vi "Periodic Tasks.vi"(8 "error in":errorcluster) -> ()   [LabVIEW 2012]
doc: "This VI runs in parallel to other tasks. It can contain as many user-defined periodic loops as you need. These can carry out PID or other sorts of timed response."
uses:
  <vilib>/Rock Robotics/SystemInterfaces/Utilities/FPGA_UtilitiesLED Source.ctl
  <vilib>/Rock Robotics/SystemInterfaces/Utilities/FPGA_UtilitiesLED State.ctl
  <vilib>/Rock Robotics/WPI/Solenoid/WPI_SolenoidValue.ctl
  <vilib>/Rock Robotics/WPI/RobotDrive/WPI_RobotDriveGetSetRefNum.vi
  <vilib>/Rock Robotics/WPI/Compressor/WPI_CompressorGetSetRefNum.vi
  Robot Global Data.vi
  <vilib>/Rock Robotics/WPI/Joystick/WPI_JoystickGetSetRefNum.vi
  <vilib>/Rock Robotics/WPI/Solenoid/WPI_SolenoidSetEnum.vi
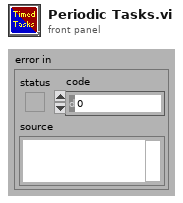
[diagram p1: front panel]
types:
  T1 = typedef "WPI_MotorControlDeviceRef.ctl" = cluster{"DeviceStatus":errorcluster, "Type":enum16{"PWM", "CAN"}, "PWM":cluster{"Digital Module":T2, "PWM Channel":T3, "DeadBand":T4}, "CAN":cluster{"Device Number":u8, "Control Mode":T5, "Semaphore":T6, "Max Vout":dbl}, "Invert":bool, "TransformRef":T7, "InvTransformRef":T7}
  T2 = typedef "FPGA_TypedefDigitalModule.ctl" = enum16{"Digital Module 1", "Digital Module 2"}
  T3 = typedef "FPGA_DIOPWMChannel.ctl" = enum8{"PWM 1", "PWM 2", "PWM 3", "PWM 4", "PWM 5", "PWM 6", "PWM 7", "PWM 8", "PWM 9", "PWM 10", "Invalid"}
  T4 = typedef "WPI_PWMDeadband.ctl" = cluster{"Name":string, "maxPositivePwm":i32, "minPositivePwm":i32, "centerPwm":i32, "maxNegativePwm":i32, "minNegativePwm":i32, "angularRange":u16}
  T5 = typedef "WPI_CANJaguar_ControlMode.ctl" = enum8{"Percent VBus", "Current", "Speed", "Position", "Voltage"}
  T6 = typedef "Semaphore RefNum" = refnum<k1>
  T7 = typedef "WPI_PWMTransform_ConPane.ctl" = refnum<vi>
  T8 = typedef "WPI_JoystickDevRef.ctl" = cluster{"Device":T9}
  T9 = typedef "WPI_JoystickDeviceEnum.ctl" = enum16{"USB 1", "USB 2", "USB 3", "USB 4", "Kinect 1", "Kinect 2"}
  T10 = typedef "WPI_JoystickButtonState.ctl" = cluster{"Button 1":bool, "Button 2":bool, "Button 3":bool, "Button 4":bool, "Button 5":bool, "Button 6":bool, "Button 7":bool, "Button 8":bool, "Button 9":bool, "Button 10":bool, "Button 11":bool, "Button 12":bool}
  T11 = cluster{"axis 1 (x)":dbl, "axis 2 (y)":dbl, "axis 3 (throttle)":dbl, "axis 4":dbl, "axis 5":dbl, "axis 6":dbl}
  T12 = typedef "WPI_SolenoidValue.ctl" = enum16{"Off", "On", "Forward", "Reverse"}
  T13 = typedef "WPI_SolenoidDevRef.ctl" = cluster{"DevStatus":errorcluster, "Solenoid Module":T14, "Forward Solenoid Channel":T15, "Reverse Solenoid Channel":T15}
  T14 = typedef "FPGA_TypedefSolenoidModule.ctl" = enum16{"Solenoid Module 1", "Solenoid Module 2"}
  T15 = typedef "WPI_SolenoidChannel.ctl" = enum8{"Solenoid 1", "Solenoid 2", "Solenoid 3", "Solenoid 4", "Solenoid 5", "Solenoid 6", "Solenoid 7", "Solenoid 8", "Invalid"}
  T16 = typedef "WPI_RobotDriveDevRef.ctl" = cluster{"DevStatus":errorcluster, "Motors[]":T1[], "Square Inputs":bool, "Max Output":dbl, "Isochronous":bool}
  T17 = typedef "WPI_CompressorDevRef.ctl" = cluster{"DevStatus":errorcluster, "DigitalInputDevRef":T18, "RelayDevRef":T20}
  T18 = typedef "WPI_DigitalInputDevRef.ctl" = cluster{"DevStatus":errorcluster, "DIO Channel":T19, "Digital Module":T2}
  T19 = typedef "FPGA_DIOChannel.ctl" = enum8{"DIO 1", "DIO 2", "DIO 3", "DIO 4", "DIO 5", "DIO 6", "DIO 7", "DIO 8", "DIO 9", "DIO 10", "DIO 11", "DIO 12", "DIO 13", "DIO 14", "Invalid"}
  T20 = typedef "WPI_RelayDevRef.ctl" = cluster{"DevStatus":errorcluster, "Relay Channel":T21, "Digital Module":T2, "Relay Direction":T22}
  T21 = typedef "FPGA_DIORelayChannel.ctl" = enum8{"Relay 1", "Relay 2", "Relay 3", "Relay 4", "Relay 5", "Relay 6", "Relay 7", "Relay 8", "Invalid"}
  T22 = typedef "WPI_RelayDirection.ctl" = enum16{"Both directions", "Forward only", "Reverse only"}
  T23 = typedef "WPI_DigitalOutputDevRef.ctl" = cluster{"Digital Module":T2, "DIO Channel":T19, "DevStatus":errorcluster}
  T24 = cluster{"JoystickDevRef":T8, "RobotDriveDevRef":T16}
  T25 = typedef "FPGA_UtilitiesLED State.ctl" = enum16{"Off", "On", "Toggle"}
  T26 = typedef "FPGA_UtilitiesLED Source.ctl" = enum16{"User LED", "FPGA LED"}
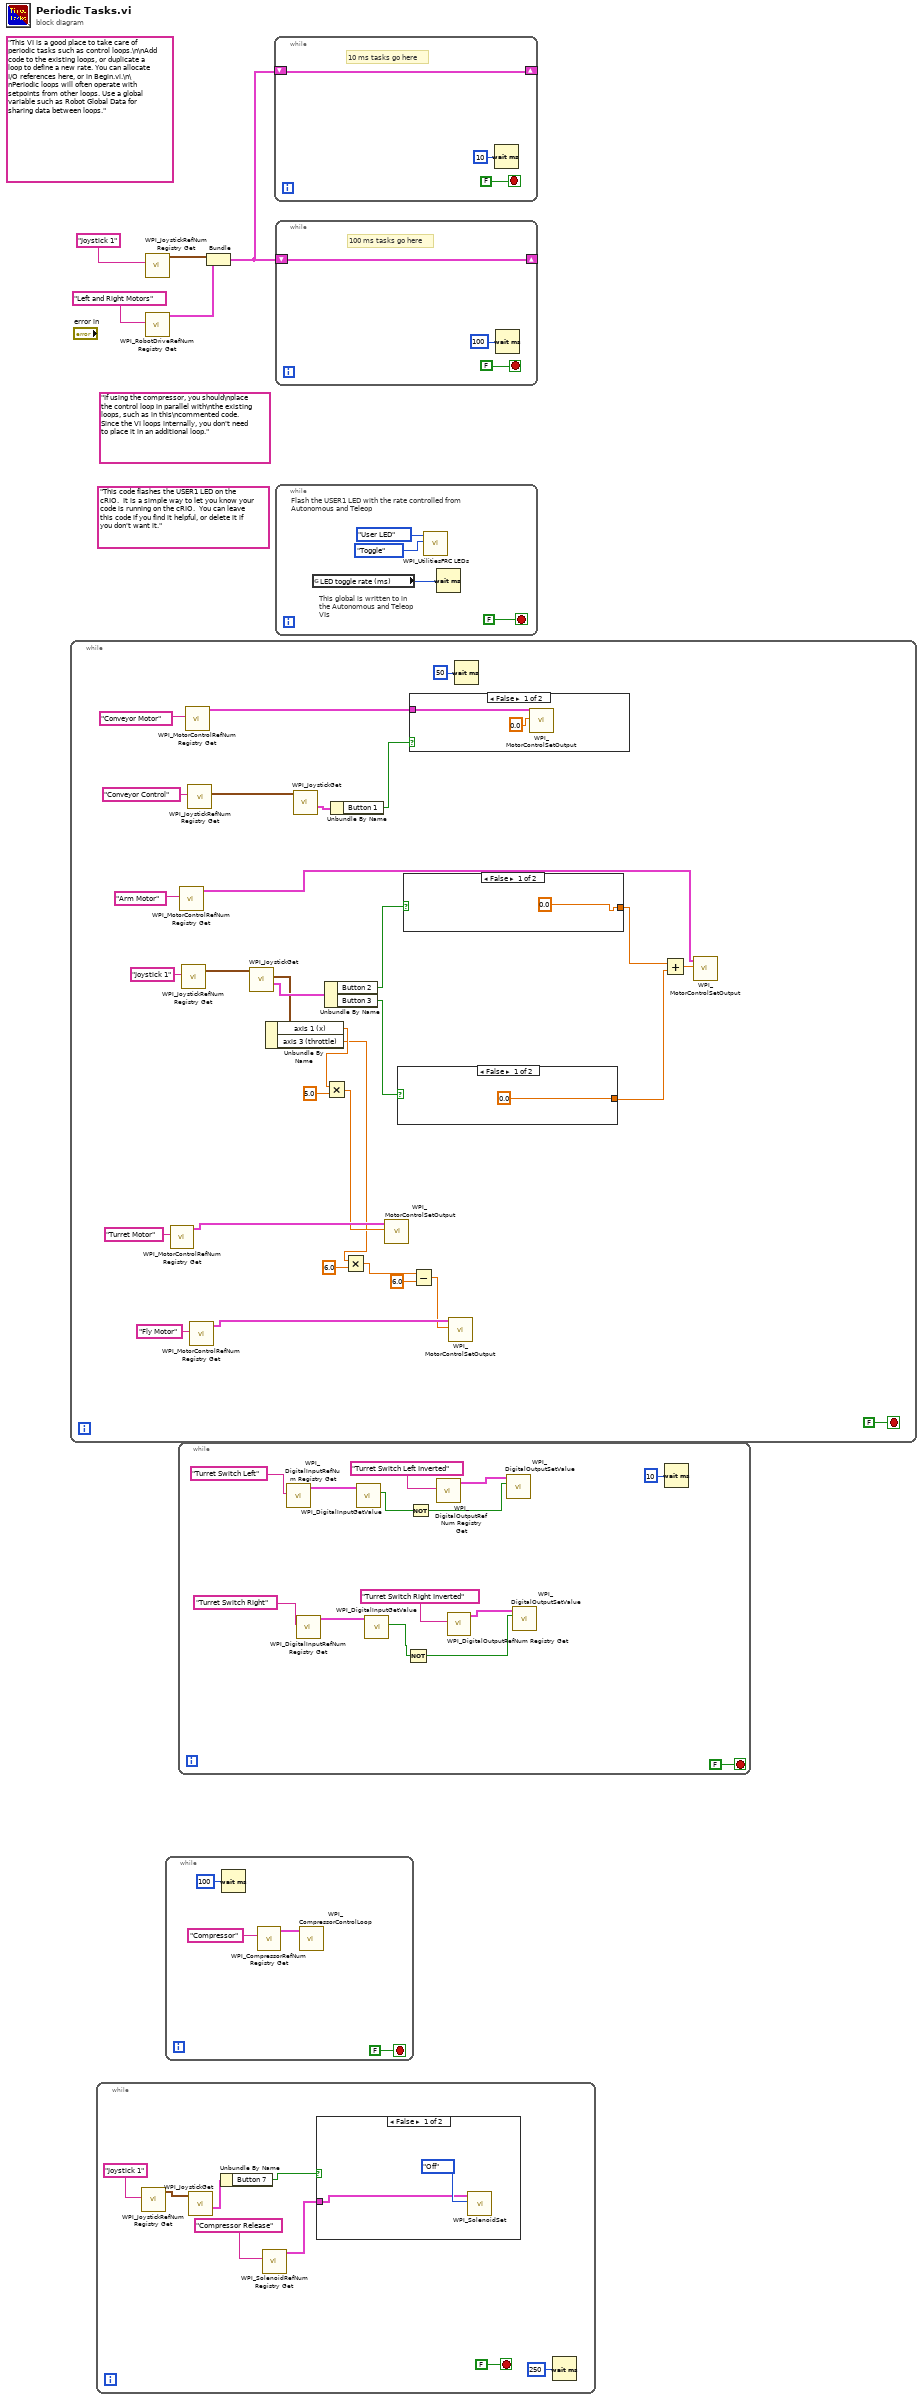
[diagram p0: block diagram]
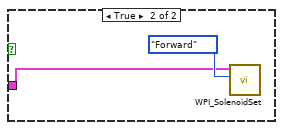
[diagram p2: hidden frame]
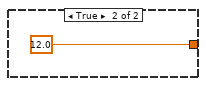
[diagram p3: hidden frame]
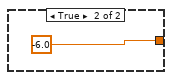
[diagram p4: hidden frame]
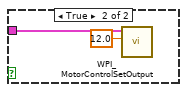
[diagram p5: hidden frame]
diagram:
  (unwired) "If using the compressor, you should\nplace the control loop in parallel with\nthe existing loops, such as in this\ncommented code. Since the VI loops internally, you don't need to place it in an additional loop."
  (unwired) "This code flashes the USER1 LED on the cRIO.  It is a simple way to let you know your code is running on the cRIO.  You can leave this code if you find it helpful, or delete it if you don't want it."
  (unwired) "This VI is a good place to take care of periodic tasks such as control loops.\n\nAdd code to the existing loops, or duplicate a loop to define a new rate. You can allocate I/O references here, or in Begin.vi.\n\nPeriodic loops will often operate with setpoints from other loops. Use a global variable such as Robot Global Data for sharing data between loops."
  n1 = while {
    stop <- FALSE stop-if-true
    n2 = call <vilib>:"WPI_MotorControlRefNum Registry Get.vi"("refnum name"="Turret Motor") -> ("MotorControlDevRef"=w20:T1)  [unwired: 9 in, 1 out]
    n3 = call <vilib>:"WPI_MotorControlRefNum Registry Get.vi"("refnum name"="Arm Motor") -> ("MotorControlDevRef"=w9:T1)  [unwired: 9 in, 1 out]
    n4 = call <vilib>:"WPI_JoystickRefNum Registry Get.vi"("refnum name"="Joystick 1") -> ("JoystickDevRef"=w26:T8)  [unwired: 9 in, 1 out]
    n5 = call <vilib>:"WPI_MotorControlRefNum Registry Get.vi"("refnum name"="Conveyor Motor") -> ("MotorControlDevRef"=w35:T1)  [unwired: 9 in, 1 out]
    n6 = call <vilib>:"WPI_JoystickRefNum Registry Get.vi"("refnum name"="Conveyor Control") -> ("JoystickDevRef"=w31:T8)  [unwired: 9 in, 1 out]
    n7 = call <vilib>:"WPI_MotorControlRefNum Registry Get.vi"("refnum name"="Fly Motor") -> ("MotorControlDevRef"=w15:T1)  [unwired: 9 in, 1 out]
    n8 = call <vilib>:"WPI_JoystickGet.vi"("JoystickDevRef"=w26) -> ("Buttons"=w25:T10, "Axes"=w21:T11)  [unwired: 4 in, 1 out]
    n9 = Unbundle By Name(w21) -> ("axis 1 (x)"=w18:dbl, "axis 3 (throttle)"=w13:dbl)
    n10 = call <vilib>:"WPI_JoystickGet.vi"("JoystickDevRef"=w31) -> ("Buttons"=w30:T10)  [unwired: 4 in, 2 out]
    n11 = Unbundle By Name(w25) -> ("Button 2"=w24:bool, "Button 3"=w23:bool)
    n12 = Multiply(x=w18, y=5.0) -> (x*y=w17:dbl)
    n13 = Unbundle By Name(w30) -> ("Button 1"=w29:bool)
    n14 = Multiply(x=w13, y=6.0) -> (x*y=w12:dbl)
    n15 = call <vilib>:"WPI_MotorControlSetOutput.vi"("Output"=w17, "MotorControlDevRef"=w20) -> ()  [unwired: 7 in, 3 out]
    n16 = case shown="False" w23 {
      tunnel: [0.0 ("Output") 12.0 ("x")] -> w6
      frame False {
      }
      frame True {
      }
    }
    n17 = case shown="False" w24 {
      tunnel: [0.0 ("x") -6.0 ("x")] -> w7
      frame False {
      }
      frame True {
      }
    }
    n18 = case shown="False" w29 {
      tunnel: w35 -> [w41 w44]
      frame False {
        n19 = call <vilib>:"WPI_MotorControlSetOutput.vi"("Output"=0.0, "MotorControlDevRef"=w41) -> ()  [unwired: 7 in, 3 out]
      }
      frame True {
        n20 = call <vilib>:"WPI_MotorControlSetOutput.vi"("Output"=12.0, "MotorControlDevRef"=w44) -> ()  [unwired: 7 in, 3 out]
      }
    }
    n21 = Subtract(x=w12, y=6.0) -> (x-y=w10:dbl)
    n22 = call <vilib>:"WPI_MotorControlSetOutput.vi"("Output"=w10, "MotorControlDevRef"=w15) -> ()  [unwired: 7 in, 3 out]
    n23 = Wait (ms)(milliseconds to wait=u32 50) -> ()  [unwired: 1 out]
    n24 = Add(x=w7, y=w6) -> (x+y=w8:dbl)
    n25 = call <vilib>:"WPI_MotorControlSetOutput.vi"("Output"=w8, "MotorControlDevRef"=w9) -> ()  [unwired: 7 in, 3 out]
  }
  n26 = while {
    stop <- FALSE stop-if-true
    n27 = call <vilib>:"WPI_JoystickRefNum Registry Get.vi"("refnum name"="Joystick 1") -> ("JoystickDevRef"=w47:T8)  [unwired: 9 in, 1 out]
    n28 = call <vilib>:"WPI_JoystickGet.vi"("JoystickDevRef"=w47) -> ("Buttons"=w46:T10)  [unwired: 4 in, 2 out]
    n29 = Unbundle By Name(w46) -> ("Button 7"=w45:bool)
    n30 = call <vilib>:"WPI_SolenoidRefNum Registry Get.vi"("refnum name"="Compressor Release") -> ("SolenoidDevRef"=w48:T13)  [unwired: 9 in, 1 out]
    n31 = case shown="False" w45 {
      tunnel: w48 -> [w53 w55]
      frame False {
        n32 = call-poly <vilib>:"WPI_SolenoidSet.vi"("Value"=WPI_SolenoidValue."Off", "SolenoidDevRef"=w53) -> ()  [unwired: 8 in, 2 out]
      }
      frame True {
        n33 = call-poly <vilib>:"WPI_SolenoidSet.vi"("Value"=WPI_SolenoidValue."Forward", "SolenoidDevRef"=w55) -> ()  [unwired: 8 in, 2 out]
      }
    }
    n34 = Wait (ms)(milliseconds to wait=u32 250) -> ()  [unwired: 1 out]
  }
  n35 = call <vilib>:"WPI_JoystickRefNum Registry Get.vi"("refnum name"="Joystick 1") -> ("JoystickDevRef"=w3:T8)  [unwired: 1 in, 9 out]
  n36 = call <vilib>:"WPI_RobotDriveRefNum Registry Get.vi"("refnum name"="Left and Right Motors") -> ("RobotDriveDevRef"=w2:T16)  [unwired: 1 in, 9 out]
  n37 = while {
    stop <- FALSE stop-if-true
    n38 = Wait (ms)(milliseconds to wait=u32 100) -> ()  [unwired: 1 out]
    n39 = call <vilib>:"WPI_CompressorRefNum Registry Get.vi"("refnum name"="Compressor") -> ("CompressorDevRef"=w60:T17)  [unwired: 9 in, 1 out]
    n40 = call <vilib>:"WPI_CompressorControlLoop.vi"("CompressorDevRef"=w60) -> ()  [unwired: 11 in]
  }
  n41 = while {
    stop <- FALSE stop-if-true
    n42 = call <vilib>:"WPI_DigitalInputRefNum Registry Get.vi"("refnum name"="Turret Switch Left") -> ("DigitalInputDevRef"=w69:T18)  [unwired: 9 in, 1 out]
    n43 = call <vilib>:"WPI_DigitalInputRefNum Registry Get.vi"("refnum name"="Turret Switch Right") -> ("DigitalInputDevRef"=w70:T18)  [unwired: 9 in, 1 out]
    n44 = call <vilib>:"WPI_DigitalInputGetValue.vi"("DigitalInputDevRef"=w69) -> ("Value"=w62:bool)  [unwired: 8 in, 2 out]
    n45 = call <vilib>:"WPI_DigitalInputGetValue.vi"("DigitalInputDevRef"=w70) -> ("Value"=w64:bool)  [unwired: 8 in, 2 out]
    n46 = Not(x=w64) -> (.not. x?=w63:bool)
    n47 = Not(x=w62) -> (.not. x?=w61:bool)
    n48 = call <vilib>:"WPI_DigitalOutputRefNum Registry Get.vi"("refnum name"="Turret Switch Left Inverted") -> ("DigitalOutputDevRef"=w65:T23)  [unwired: 9 in, 1 out]
    n49 = call <vilib>:"WPI_DigitalOutputRefNum Registry Get.vi"("refnum name"="Turret Switch Right Inverted") -> ("DigitalOutputDevRef"=w66:T23)  [unwired: 9 in, 1 out]
    n50 = call <vilib>:"WPI_DigitalOutputSetValue.vi"("Value"=w61, "DigitalOutputDevRef"=w65) -> ()  [unwired: 8 in, 2 out]
    n51 = call <vilib>:"WPI_DigitalOutputSetValue.vi"("Value"=w63, "DigitalOutputDevRef"=w66) -> ()  [unwired: 8 in, 2 out]
    n52 = Wait (ms)(milliseconds to wait=u32 10) -> ()  [unwired: 1 out]
  }
  n53 = Bundle("JoystickDevRef"=w3, "RobotDriveDevRef"=w2) -> (w1:T24)  [unwired: 1 out]
  n54 = while {
    shift-right: [w75] -> _
    shift-left: w1 -> [w75]
    stop <- FALSE stop-if-true
    # "10 ms tasks go here"
    n55 = Wait (ms)(milliseconds to wait=u32 10) -> ()  [unwired: 1 out]
  }
  n56 = while {
    shift-right: [w78] -> _
    shift-left: w1 -> [w78]
    stop <- FALSE stop-if-true
    # "100 ms tasks go here"
    n57 = Wait (ms)(milliseconds to wait=u32 100) -> ()  [unwired: 1 out]
  }
  n58 = while {
    stop <- FALSE stop-if-true
    # "This global is written to in the Autonomous and Teleop VIs"
    # "Flash the USER1 LED with the rate controlled from Autonomous and Teleop"
    n59 = global read "Robot Global Data.vi" "LED toggle rate (ms)"() -> (w81:u32)
    n60 = call <vilib>:"WPI_UtilitiesFRC LEDs.vi"("State"=FPGA_UtilitiesLED_State."Toggle", "LED Type"=FPGA_UtilitiesLED_Source."User LED") -> ()  [unwired: 1 in, 9 out]
    n61 = Wait (ms)(milliseconds to wait=w81) -> ()  [unwired: 1 out]
  }
